vi "Register for Broadcast Events.vi"(8 "error in (no error)":errorcluster, 11 "Asynchronous Action In":refnum<class "Asynchronous Action.lvclass">) -> (0 "error out":errorcluster, 2 "Event Registration Refnum":refnum<event-registration>, 3 "Asynchronous Action Out":refnum<class "Asynchronous Action.lvclass">)   [LabVIEW 2020, in "Asynchronous Action.lvclass"]
doc: "Returns a registration to broadcase messages from the process and any owned processes."
uses:
  Asynchronous Action.lvclass
  Process/Protected/Broadcasting/Broadcast Message Cluster.ctl
  Process/Process.lvclass
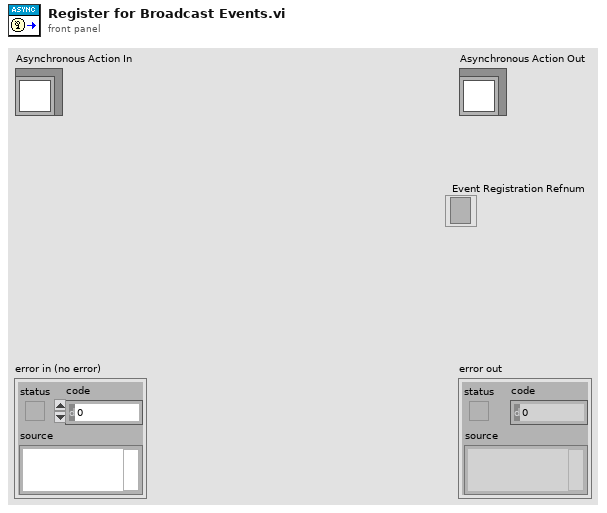
[diagram p1: front panel]
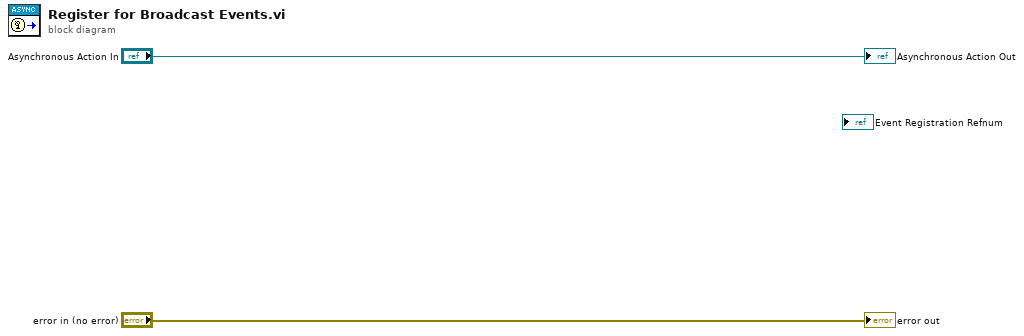
[diagram p0: block diagram]
diagram:
  "error out" <- "error in (no error)"
  "Asynchronous Action Out" <- "Asynchronous Action In"
